vi "encoder_test.vi"() -> ()   [LabVIEW 2014]
uses:
  <vilib>/rvi/FXPMathLib/FxpSinAndCos/subVIs/nifxpmath_SinAndCos_SimConfig.ctl
  <vilib>/rvi/Emulation/niFpgaGetClockAttributes.vi
  <vilib>/rvi/Emulation/niFpgaSctlEmulationGetInTimedLoop.vi
  <vilib>/rvi/Emulation/niFpgaEmulationReportErrorSimple.vi
  <vilib>/rvi/eio/common/nirviEmuTemplateMethod_errors.vi
  <vilib>/rvi/Emulation/niFpgaProcessEmulError.vi
  <vilib>/rvi/Emulation/niFpgaCriticalErrorInLSC.vi
  <vilib>/rvi/FXPMathLib/FxpSinAndCos/simVIs/DllFxpSinAndCosTemp_sub.vi
  <vilib>/rvi/interface/RandomDataEmulation/nirviRandomDataMultiElementFPGAFIFO.vi
  <instcachedir>/0/nirviRandomDataMultiElementFPGAFIFO_AD0CFC12EF974623A9C2E4184BC062B2.lvgen/nirviRandomDataMultiElementFPGAFIFO_AD0CFC12EF974623A9C2E4184BC062B2_020.vi
  <vilib>/rvi/interface/RandomDataEmulation/niFpgaRandomDataHandleErrors.vi
  <vilib>/eio/EIONode/EIONode.xnode
  <vilib>/rvi/FXPMathLib/FxpMul/XNode/nifxpmath_Multiplier.xnode
  <vilib>/rvi/FXPMathLib/FxpSinAndCos/XNode/nifxpmath_SinAndCos.xnode
  <vilib>/rvi/Analysis/measure/butterworth/XNode/niFpgaButterworthFilter.xnode
  <vilib>/rvi/FXPMathLib/FxpSub/XNode/nifxpmath_Sub.xnode
  <vilib>/rvi/FXPMathLib/FxpAdd/XNode/nifxpmath_Add.xnode
  <vilib>/rvi/DataTransferAndStorage/Container/XNode/niFpgaContainer.xnode
  <vilib>/rvi/interface/RandomDataEmulation/nirviRandomDataFpgaMultiElementTemplate.vi
  <vilib>/rvi/FXPMathLib/sim/FxpSim.dll
panel:
  out "D_i":fxp<+/-,34,18>
  in  "D_tolorence":fxp<+/-,14,3>
  in  "Ki":fxp<+/-,20,6>
  out "D_error":fxp<+/-,24,11>
  in  "Direction":bool
  out "Fmr_PD":fxp<+/-,64,31>
  in  "Kd":fxp<+/-,20,8>
  in  "Dr":fxp<+/-,11,7>
  in  "Kp":fxp<+/-,20,12>
  in  "scaled coefficients_D_dd":i32[](array[numeric])=[780119100, 146811362]
  out "D_dd":fxp<+/-,36,29>
  in  "Ini coe.":bool
  out "va":fxp<+/-,38,8>
  out "vb":fxp<+/-,38,8>
  in  "stop motor":bool
  out "vq_F":fxp<+/-,20,5> format="%.57g"
  out "vd_F":fxp<+/-,20,5>
  out "D_d (mm/s)":fxp<+/-,32,12>
  out "mt":u32
  out "omega (rad/s)":fxp<+/-,32,18>
  in  "mt0":u32
  out "D(mm)":fxp<+/-,22,7>
  out "rad(NrTheta)":fxp<+/-,33,18>
  out "Encoder Position":i32
  in  "Encoder Reset":bool
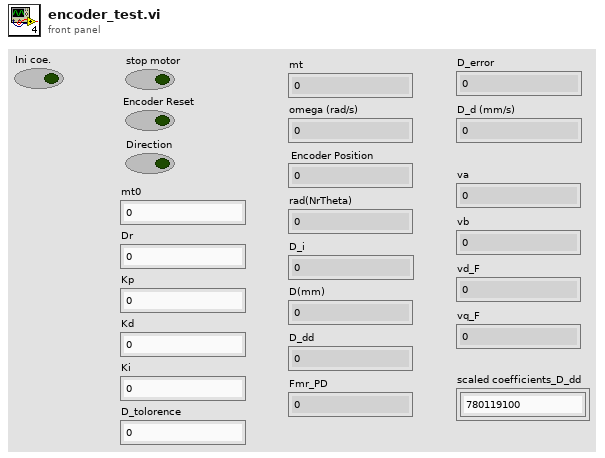
[diagram p1: front panel]
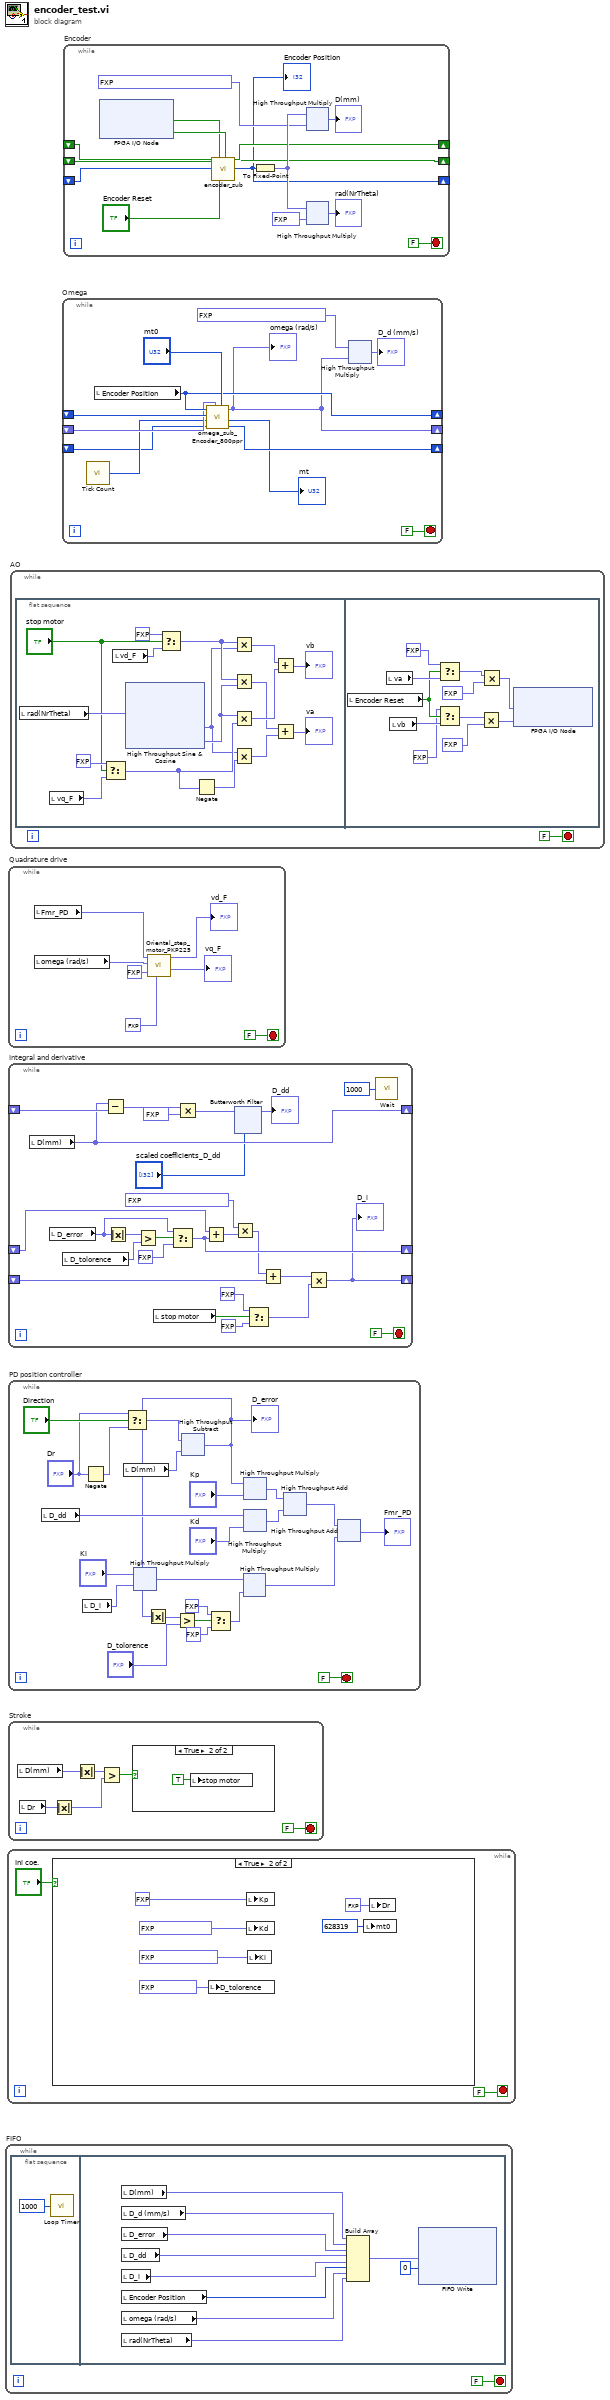
[diagram p0: block diagram]
diagram:
  n1 = while "FIFO" {
    stop <- FALSE stop-if-true
    n2 = flat-sequence {
      frame #0 {
        n3 = call "Loop Timer"("Count(uSec)"=u32 1000) -> ()  [unwired: 1 out]
      }
      frame #1 {
        n4 = local read "D(mm)"() -> (w10:fxp<+/-,22,7>)
        n5 = local read "D_d (mm/s)"() -> (w9:fxp<+/-,32,12>)
        n6 = local read "D_error"() -> (w8:fxp<+/-,24,11>)
        n7 = local read "D_dd"() -> (w7:fxp<+/-,36,29>)
        n8 = local read "D_i"() -> (w6:fxp<+/-,34,18>)
        n9 = local read "Encoder Position"() -> (w5:i32)
        n10 = local read "omega (rad/s)"() -> (w4:fxp<+/-,32,18>)
        n11 = local read "rad(NrTheta)"() -> (w3:fxp<+/-,33,18>)
        n12 = Build Array(w10, w9, w8, w7, w6, w5, w4, w3) -> (w11:fxp<+/-,52,32>[])
        n13 = xnode ("FIFO Write")("Element"=w11, "Timeout"=0) -> ()  [unwired: 1 in, 2 out]
      }
    }
  }
  n14 = while {
    stop <- FALSE stop-if-true
    n15 = case shown="True" "Ini coe." {
      frame False {
      }
      frame True {
        n16 = local write "D_tolorence"(fxp<+/-,14,3> 0.009765625 ("D_tolorence")) -> ()
        n17 = local write "Kp"(fxp<+/-,20,12> 2.0 ("Kp")) -> ()
        n18 = local write "Kd"(fxp<+/-,20,8> 1.800048828125 ("Kd")) -> ()
        n19 = local write "Ki"(fxp<+/-,20,6> 0.0999755859375 ("D_i")) -> ()
        n20 = local write "mt0"(u32 628319 ("mt0")) -> ()
        n21 = local write "Dr"(fxp<+/-,11,7> 20.0 ("Fmr")) -> ()
      }
    }
  }
  n22 = while "Quadrature drive" {
    stop <- FALSE stop-if-true
    n23 = local read "Fmr_PD"() -> (w21:fxp<+/-,64,31>)
    n24 = local read "omega (rad/s)"() -> (w23:fxp<+/-,32,18>)
    n25 = call "Oriental_step_motor_PKP225.vi"("F_Threshold"=fxp<+,12,12> 10.0, "dFmr"=fxp<+/-,25,15> 0.0, "omega"=w23, "Fmr"=w21) -> ("vq_F"=→"vq_F":fxp<+/-,20,5>, "vd_F"=→"vd_F":fxp<+/-,20,5>)  [unwired: 6 in]
  }
  n26 = while "Integral and derivative" {
    shift-right: [w48] -> _
    shift-left: _ -> [w52]
    shift-right: [w38] -> _
    shift-left: _ -> [w39]
    shift-right: [w28] -> _
    shift-left: _ -> [w32]
    stop <- FALSE stop-if-true
    n27 = local read "D(mm)"() -> (w48:fxp<+/-,22,7>)
    n28 = local read "D_error"() -> (w40:fxp<+/-,24,11>)
    n29 = local read "D_tolorence"() -> (w43:fxp<+/-,14,3>)
    n30 = Subtract(x=w48, y=w52) -> (x-y=w51:fxp<+/-,23,8>)
    n31 = Absolute Value(x=w40) -> (abs(x)=w44:fxp<+,24,11>)
    n32 = Greater?(x=w44, y=w43) -> (0:w42:bool)
    n33 = local read "stop motor"() -> (w35:bool)
    n34 = Select(t=w40, s=w42, f=fxp<+,24,11> 0.0) -> (s? t:f=w38:fxp<+/-,25,12>)
    n35 = Multiply(x=w51, y=fxp<+/-,33,13> 1000.0) -> (x*y=w49:fxp<+/-,55,20>)
    n36 = Add(x=w39, y=w38) -> (x+y=w37:fxp<+/-,26,13>)
    n37 = Multiply(x=fxp<+/-,30,12> 0.000499725341796875, y=w37) -> (x*y=w31:fxp<+/-,55,24>)
    n38 = xnode "Butterworth Filter"("input data"=w49, "scaled coefficients"="scaled coefficients_D_dd") -> ("output data"=→"D_dd":fxp<+/-,36,24>)  [unwired: 1 in]
    n39 = Select(t=fxp<+,1,1> 0.0, s=w35, f=fxp<+,1,1> 1.0) -> (s? t:f=w29:fxp<+,1,1>)
    n40 = Add(x=w31, y=w32) -> (x+y=w30:fxp<+/-,32,16>)
    n41 = Multiply(x=w30, y=w29) -> (x*y=w28:fxp<+/-,32,16>)
    "D_i" <- w28
    n42 = call "Wait"("Count(uSec)"=u32 1000) -> ()  [unwired: 1 out]
  }
  n43 = while "PD position controller" {
    stop <- FALSE stop-if-true
    n44 = local read "D_dd"() -> (w81:fxp<+/-,36,29>)
    n45 = local read "D_i"() -> (w72:fxp<+/-,34,18>)
    n46 = Negate(x="Dr") -> (-x=w76:fxp<+/-,12,8>)
    n47 = local read "D(mm)"() -> (w85:fxp<+/-,22,7>)
    n48 = Select(t="Dr", s="Direction", f=w76) -> (s? t:f=w75:fxp<+/-,12,8>)
    n49 = xnode ("High Throughput Multiply")("x"="Ki", "y"=w72) -> ("x*y"=w66:fxp<+/-,54,24>)
    n50 = xnode "High Throughput Subtract"("x"=w75, "y"=w85) -> ("x-y"=w70:fxp<+/-,24,9>)
    "D_error" <- w70
    n51 = Absolute Value(x=w70) -> (abs(x)=w71:fxp<+,24,9>)
    n52 = Greater?(x=w71, y="D_tolorence") -> (0:w69:bool)
    n53 = Select(t=fxp<+,10,2> 1.0, s=w69, f=fxp<+,10,2> 0.0) -> (s? t:f=w65:fxp<+,10,2>)
    n54 = xnode ("High Throughput Multiply")("x"=w66, "y"=w65) -> ("x*y"=w62:fxp<+/-,64,26>)
    n55 = xnode ("High Throughput Multiply")("x"=w70, "y"="Kp") -> ("x*y"=w83:fxp<+/-,44,21>)
    n56 = xnode ("High Throughput Multiply")("x"=w81, "y"="Kd") -> ("x*y"=w82:fxp<+/-,56,37>)
    n57 = xnode ("High Throughput Add")("x"=w83, "y"=w82) -> ("x+y"=w63:fxp<+/-,61,38>)
    n58 = xnode ("High Throughput Add")("x"=w63, "y"=w62) -> ("x+y"=→"Fmr_PD":fxp<+/-,64,39>)
  }
  n59 = while "Stroke" {
    stop <- FALSE stop-if-true
    n60 = local read "D(mm)"() -> (w91:fxp<+/-,22,7>)
    n61 = local read "Dr"() -> (w87:fxp<+/-,11,7>)
    n62 = Absolute Value(x=w87) -> (abs(x)=w86:fxp<+,11,7>)
    n63 = Absolute Value(x=w91) -> (abs(x)=w90:fxp<+,22,7>)
    n64 = Greater?(x=w90, y=w86) -> (0:w89:bool)
    n65 = case shown="True" w89 {
      frame False {
      }
      frame True {
        n66 = local write "stop motor"(TRUE ("stop motor")) -> ()
      }
    }
  }
  n67 = while "AO" {
    stop <- FALSE stop-if-true
    n68 = flat-sequence {
      frame #0 {
        n69 = local read "rad(NrTheta)"() -> (w109:fxp<+/-,33,18>)
        n70 = local read "vq_F"() -> (w107:fxp<+/-,20,5>)
        n71 = Select(t=fxp<+,20,5> 0.0, s="stop motor", f=w107) -> (s? t:f=w104:fxp<+/-,21,6>)
        n72 = local read "vd_F"() -> (w108:fxp<+/-,20,5>)
        n73 = xnode "High Throughput Sine & Cosine"("x (pi)"=w109) -> ("sin(x)"=w100:fxp<+/-,17,2>, "cos(x)"=w102:fxp<+/-,17,2>)
        n74 = Select(t=fxp<+,20,5> 0.0, s="stop motor", f=w108) -> (s? t:f=w101:fxp<+/-,21,6>)
        n75 = Negate(x=w104) -> (-x=w103:fxp<+/-,21,6>)
        n76 = Multiply(x=w101, y=w100) -> (x*y=w99:fxp<+/-,37,7>)
        n77 = Multiply(x=w101, y=w102) -> (x*y=w97:fxp<+/-,37,7>)
        n78 = Multiply(x=w102, y=w104) -> (x*y=w98:fxp<+/-,37,7>)
        n79 = Multiply(x=w100, y=w103) -> (x*y=w96:fxp<+/-,37,7>)
        n80 = Add(x=w99, y=w98) -> (x+y=→"vb":fxp<+/-,38,8>)
        n81 = Add(x=w97, y=w96) -> (x+y=→"va":fxp<+/-,38,8>)
      }
      frame #1 {
        n82 = local read "Encoder Reset"() -> (w143:bool)
        n83 = local read "va"() -> (w145:fxp<+/-,38,8>)
        n84 = local read "vb"() -> (w144:fxp<+/-,38,8>)
        n85 = Select(t=fxp<+/-,20,5> 5.0 ("y"), s=w143, f=w145) -> (s? t:f=w146:fxp<+/-,38,8>)
        n86 = Select(t=fxp<+/-,20,5> 0.0 ("y"), s=w143, f=w144) -> (s? t:f=w147:fxp<+/-,38,8>)
        n87 = Multiply(x=w147, y=fxp<+/-,20,5> -0.5) -> (x*y=w151:fxp<+/-,57,12>)
        n88 = Multiply(x=w146, y=fxp<+/-,20,5> -0.5) -> (x*y=w150:fxp<+/-,57,12>)
        n89 = xnode "FPGA I/O Node"("Mod8/AO0"=w150, "Mod8/AO1"=w151) -> ()  [unwired: 2 in, 2 out]
      }
    }
  }
  n90 = while "Omega" {
    shift-right: [w161] -> _
    shift-left: _ -> [w162]
    shift-right: [w154] -> _
    shift-left: _ -> [w160]
    shift-right: [w157] -> _
    shift-left: _ -> [w158]
    stop <- FALSE stop-if-true
    n91 = call "Tick Count"() -> ("Tick Count(Ticks)"=w159:u32)
    n92 = local read "Encoder Position"() -> (w161:i32)
    n93 = call "omega_sub_Encoder_800ppr.vi"("mt0"="mt0", "omega_pre"=w160, "ticks_m_pre"=w158, "ticks"=w159, "count_pre"=w162, "count"=w161) -> ("ticks_m"=w157:u32, "mt"=→"mt":u32, "omega"=w154:fxp<+/-,20,9>)  [unwired: 3 in]
    "omega (rad/s)" <- w154
    n94 = xnode ("High Throughput Multiply")("x"=fxp<+/-,26,1> 0.3183099031448364, "y"=w154) -> ("x*y"=→"D_d (mm/s)":fxp<+/-,46,10>)
  }
  n95 = while "Encoder" {
    shift-right: [w170] -> _
    shift-left: _ -> [w172]
    shift-right: [w169] -> _
    shift-left: _ -> [w171]
    shift-right: [w167] -> _
    shift-left: _ -> [w168]
    stop <- FALSE stop-if-true
    n96 = xnode "FPGA I/O Node"() -> ("Mod4/DI3"=w177:bool, "Mod4/DI4"=w178:bool)  [unwired: 2 in, 2 out]
    n97 = call "encoder_sub.vi"("A_pre"=w172, "B_pre"=w171, "Encoder Position_pre"=w168, "A input"=w177, "Encoder Position Reset"="Encoder Reset", "B input"=w178) -> ("A"=w170:bool, "B"=w169:bool, "Encoder Position (Counts)"=w167:i32)  [unwired: 19 in]
    "Encoder Position" <- w167
    n98 = To Fixed-Point(number=w167) -> (fixed-point=w175:fxp<+/-,32,32>)  [unwired: 1 in]
    n99 = xnode ("High Throughput Multiply")("x"=w175, "y"=fxp<+/-,24,0> 0.002499997615814209) -> ("x*y"=→"D(mm)":fxp<+/-,56,32>)
    n100 = xnode ("High Throughput Multiply")("x"=w175, "y"=fxp<+/-,24,0> 0.125) -> ("x*y"=→"rad(NrTheta)":fxp<+/-,56,32>)
  }
